vi "Amplitude and Levels 1 chan (obs).vi"(6 "state settings":T1={"method"=enum."auto select", "histogram size"=256, "histogram method"=enum."mode", "reserved"=1.0} {"reserved" format="%0.2f"}, 8 "error in (no error)":errorcluster, 11 "signal in":waveform(dbl)) -> (0 "error out":errorcluster, 1 "low state level":dbl format="%.2g", 2 "high state level":dbl format="%.2g", 3 "amplitude":dbl format="%.2p")   [LabVIEW 2020, in "NI_MAPro.lvlib"]
uses:
  NI_MAPro.lvlib
  <resource>/lvanlys.dll
  NI_MABase.lvlib
panel:
  # "This VI is obsolete !!!\nYou should replace this VI in your diagram with the Amplitude and Levels VI."
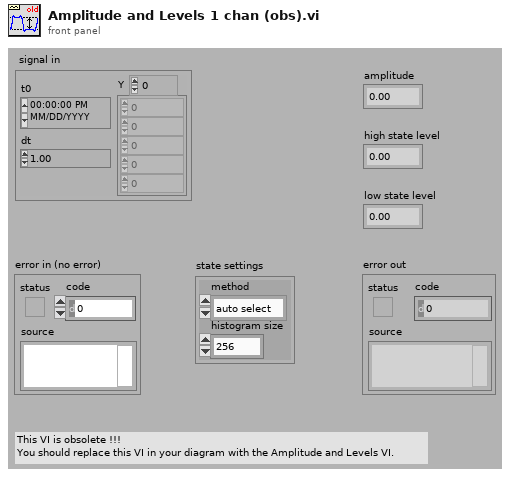
[diagram p1: front panel]
types:
  T1 = cluster{"method":enum32{"histogram", "peak", "auto select"}, "histogram size":i32, "histogram method":enum16{"mode"}, "reserved":dbl}
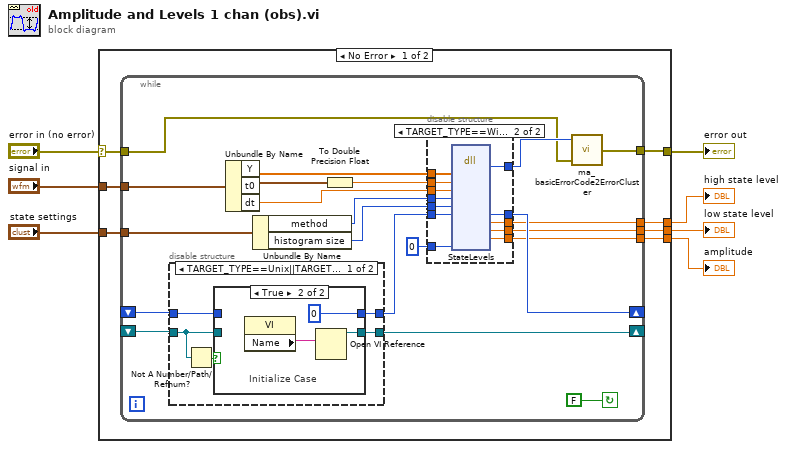
[diagram p0: block diagram]
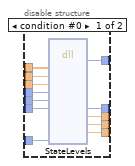
[diagram p2: hidden frame]
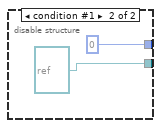
[diagram p4: hidden frame]
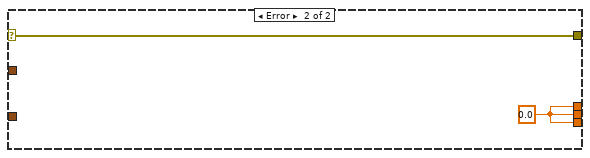
[diagram p5: hidden frame]
diagram:
  n1 = case shown="No Error" "error in (no error)" {
    selector: "error in (no error)" -> [w9 w73]
    tunnel: [w8 w73] -> w1
    tunnel: "signal in" -> [w14 _]
    tunnel: "state settings" -> [w13 _]
    tunnel: [w12 w72] -> w4
    tunnel: [w11 w72] -> w3
    tunnel: [w10 w72] -> w2
    frame No Error {
      n2 = while {
        shift-left: _ -> [w22]
        shift-right: [w26] -> _
        shift-right: [w19] -> _
        shift-left: _ -> [w21]
        tunnel: w14 -> [w28]
        tunnel: w13 -> [w27]
        tunnel: [w16] -> w8
        tunnel: [w25] -> w12
        tunnel: [w24] -> w11
        tunnel: [w23] -> w10
        tunnel: w9 -> [w15]
        stop <- FALSE continue-if-true
        n3 = disable-structure shown="TARGET_TYPE==Unix||TARGET_TYPE==Mac||TARGET_TYPE==RT||TARGET_TYPE==Windows, Default" {
          disable-tunnel: w21 -> [w62 _]
          disable-tunnel: [w63 refnum<vi> refnum ("VI Refnum")] -> w19
          disable-tunnel: w22 -> [w61 _]
          disable-tunnel: [w60 0 ("t")] -> w20
          frame condition #0 (active) {
            n4 = Not A Number/Path/Refnum?(number/path/refnum=w62) -> (NaN/Path/Refnum?=w64:bool)
            n5 = case shown="True" w64 {
              tunnel: [w66 w68] -> w63
              tunnel: w62 -> [w66 _]
              tunnel: w61 -> [w65 _]
              tunnel: [w65 0 ("error")] -> w60
              frame False {
              }
              frame True {
                # "Initialize Case"
                n6 = property class="VI"() -> ("Name"=w67:string)  [unwired: 2 in, 2 out]
                n7 = Open VI Reference(vi path=w67) -> (vi reference=w68:refnum<vi>)  [unwired: 1 in, 5 out]
              }
            }
          }
          frame condition #1 {
          }
        }
        n8 = Unbundle By Name(w28) -> ("Y"=w29:dbl[], "t0"=w32:timestamp, "dt"=w34:dbl)
        n9 = Unbundle By Name(w27) -> ("method"=w31:enum32{"histogram", "peak", "auto select"}, "histogram size"=w30:i32)
        n10 = To Double Precision Float(number=w32) -> (double precision float=w33:dbl)
        n11 = disable-structure shown="TARGET_TYPE==Windows||TARGET_TYPE==Mac||TARGET_TYPE==Unix||TARGET_BITNESS==64" {
          disable-tunnel: w34 -> [w47 w59]
          disable-tunnel: w33 -> [w46 w58]
          disable-tunnel: w31 -> [w45 w57]
          disable-tunnel: w30 -> [w44 w56]
          disable-tunnel: [w43 w55] -> w17
          disable-tunnel: w29 -> [w42 w54]
          disable-tunnel: [w41 w53] -> w26
          disable-tunnel: [w40 w52] -> w25
          disable-tunnel: [w39 w51] -> w24
          disable-tunnel: [w38 w50] -> w23
          disable-tunnel: w20 -> [w37 w49]
          disable-tunnel: 0 ("newAlgorithm") -> [w36 w48]
          frame condition #0 {
            n12 = dll-call lib="C:/Program Files (x86)/National Instruments/LabVIEW 2020/resource/lvanlys.*" fn="StateLevels"("xH"=w42, "Xo"=w46, "dx"=w47, "method"=w45, "histoSize"=w44, "work"=w37, "newAlgorithm"=w36) -> ("return type"=w43:i32, "work"=w41:i32, "high"=w40:dbl, "low"=w39:dbl, "amp"=w38:dbl)  [unwired: 12 in, 2 out]
          }
          frame condition #1 (active) {
            n13 = dll-call lib="C:/Program Files (x86)/National Instruments/LabVIEW 2020/resource/lvanlys.dll" fn="StateLevels"("xH"=w54, "Xo"=w58, "dx"=w59, "method"=w57, "histoSize"=w56, "work"=w49, "newAlgorithm"=w48) -> ("return type"=w55:i32, "work"=w53:i64, "high"=w52:dbl, "low"=w51:dbl, "amp"=w50:dbl)  [unwired: 8 in, 6 out]
          }
        }
        n14 = call "ma_basicErrorCode2ErrorCluster.vi"("error in (no error)"=w15, "Error Code"=w17) -> ("error out"=w16:errorcluster)  [unwired: 1 in]
      }
    }
    frame Error {
      w72 = 0.0 ("high")
    }
  }
  "amplitude" <- w2
  "low state level" <- w3
  "error out" <- w1
  "high state level" <- w4
